vi "Create.vi"(8 "error in (no error)":errorcluster, 9 "Config Path":path, 10 "Config Module":refnum<class "MessageQ.lvclass">) -> (0 "error out":errorcluster, 3 "ConfigHTTPController out":refnum<class "ConfigHTTPController.lvclass">)   [LabVIEW 2020, in "Volatus.lvlib" / "ConfigHTTPController.lvclass"]
uses:
  ConfigHTTPController.lvclass
  MessageQ/MessageQ.lvclass
  ConfigHTTPController.lvclass/ConfigHTTPController.ctl
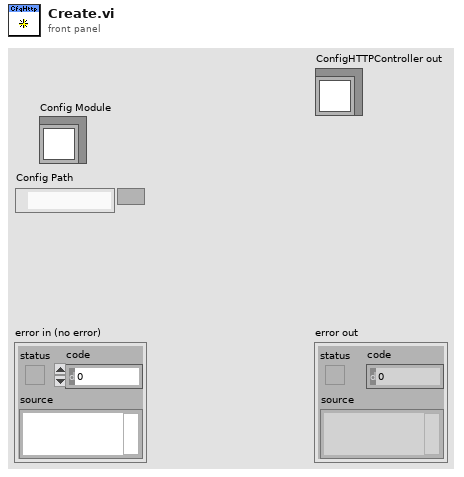
[diagram p1: front panel]
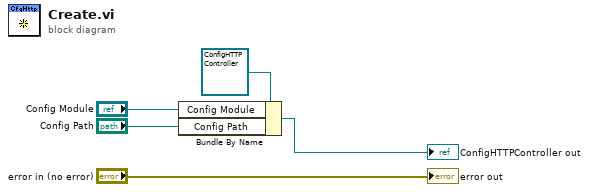
[diagram p0: block diagram]
diagram:
  n1 = Bundle By Name(cluster=refnum<class "ConfigHTTPController.lvclass"> refnum ("ConfigHTTPController in"), "Config Module"="Config Module", "Config Path"="Config Path") -> (→"ConfigHTTPController out":refnum<class "ConfigHTTPController.lvclass">)
  "error out" <- "error in (no error)"
